vi "Get SimulationFlag.vi"(8 "error in (no error)":errorcluster, 11 "Device in":refnum<class "DAQ_Device.lvclass">) -> (0 "error out":errorcluster, 2 "Simulation?":bool, 3 "Device out":refnum<class "DAQ_Device.lvclass">)   [LabVIEW 2023, in "DAQ_Device.lvclass"]
uses:
  DAQ_Device.lvclass
  DAQ_Device.lvclass/DAQ_Device.ctl
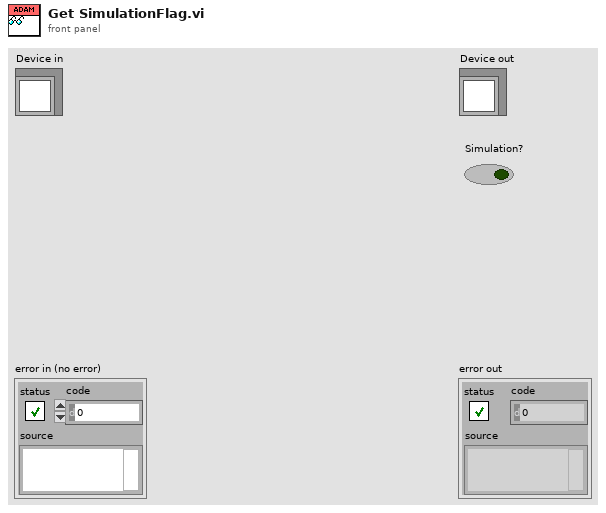
[diagram p1: front panel]
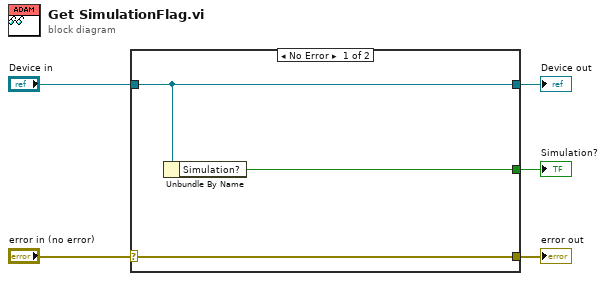
[diagram p0: block diagram]
diagram:
  n1 = case shown="No Error" "error in (no error)" {
    selector: "error in (no error)" -> [w8 w9]
    tunnel: [w8 w9] -> w4
    tunnel: [w7 w10] -> w2
    tunnel: "Device in" -> [w7 w10]
    tunnel: [w6 _] -> w1
    frame No Error {
      n2 = Unbundle By Name(w7) -> ("Simulation?"=w6:bool)
    }
    frame Error {
    }
  }
  "error out" <- w4
  "Device out" <- w2
  "Simulation?" <- w1
